vi "Master_CAN.vi"(8 "error in":errorcluster) -> (0 "error out":errorcluster)   [LabVIEW 2018]
uses:
  Control/TypeDef_DigitalOuts.ctl
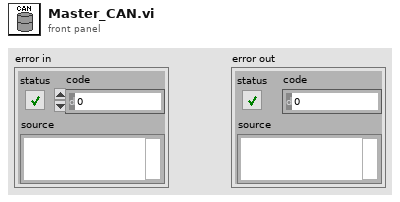
[diagram p1: front panel]
types:
  T1 = typedef "TypeDef_DigitalOuts.ctl" = cluster{"Pod Power":bool, "Dump Valve":bool, "Brakes":bool, "Clamp":bool, "Pump":bool, "Ignition":bool, "DO6":bool, "DO7":bool, "HighSide":bool, "Precharge":bool, "LowSide":bool, "DO3":bool, "DO4":bool, "DO5":bool, "DO62":bool, "DO72":bool}
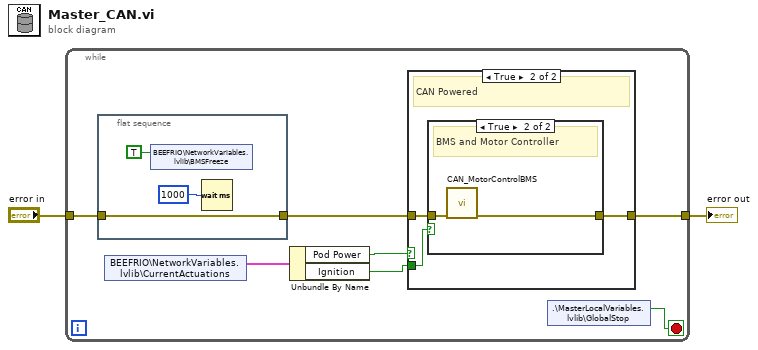
[diagram p0: block diagram]
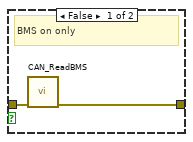
[diagram p3: hidden frame]
diagram:
  n1 = while {
    tunnel: "error in" -> [w8]
    tunnel: [w9] -> w1
    stop <- w5 stop-if-true
    n2 = flat-sequence {
      tunnel: [w19] -> w7
      tunnel: w8 -> [w19]
      frame #0 {
        n3 = shared-variable "BEEFRIO\\NetworkVariables.lvlib\\BMSFreeze"(TRUE ("BMSFreeze")) -> ()  [unwired: 1 in, 1 out]
        n4 = Wait (ms)(milliseconds to wait=u32 1000) -> ()  [unwired: 1 out]
      }
    }
    n5 = shared-variable "BEEFRIO\\NetworkVariables.lvlib\\CurrentActuations"() -> (w6:T1)  [unwired: 1 in, 1 out]
    n6 = Unbundle By Name(w6) -> ("Pod Power"=w4:bool, "Ignition"=w3:bool)
    n7 = case shown="True" w4 {
      tunnel: [w10 w13] -> w9
      tunnel: w7 -> [w10 w12]
      tunnel: w3 -> [_ w11]
      frame False {
      }
      frame True {
        # "CAN Powered"
        n8 = case shown="True" w11 {
          tunnel: [w14 w17] -> w13
          tunnel: w12 -> [w15 w16]
          frame False {
            # "BMS on only"
            n9 = call "CAN_ReadBMS.vi"("error in (no error)"=w15) -> ("error out"=w14:errorcluster)  [unwired: 10 in]
          }
          frame True {
            # "BMS and Motor Controller"
            n10 = call "CAN_MotorControlBMS.vi"("error in (no error)"=w16) -> ("error out"=w17:errorcluster)  [unwired: 10 in]
          }
        }
      }
    }
    n11 = shared-variable ".\\MasterLocalVariables.lvlib\\GlobalStop"() -> (w5:bool)  [unwired: 1 in, 1 out]
  }
  "error out" <- w1
